vi "Job.BuildSpec_BuildSpecification.vi"(8 "error in (no error)":errorcluster, 11 "Job.BuildSpec in":refnum<class "Job.BuildSpec.lvclass">) -> (0 "error out":errorcluster, 3 "Job.BuildSpec out":refnum<class "Job.BuildSpec.lvclass">)   [LabVIEW 2013, in "Job.BuildSpec.lvclass"]
uses:
  Job.BuildSpec.lvclass
  Job.BuildSpec.lvclass/Job.BuildSpec.ctl
  <vilib>/AppBuilder/AB_API_Simple/Build (path).vi
  <vilib>/LabVIEW Open Source Project/Cron Scheduler/Job/Job.lvclass
  <vilib>/AppBuilder/AB_API_Simple/NI_App_Builder_API.lvlib
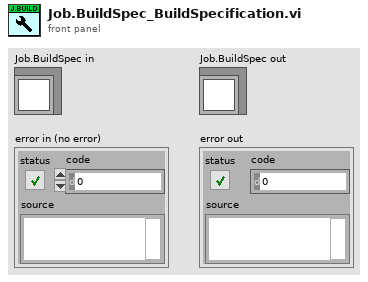
[diagram p1: front panel]
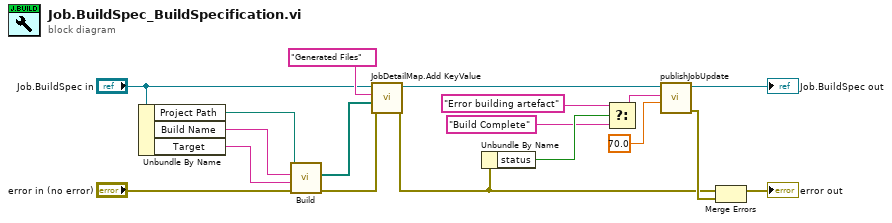
[diagram p0: block diagram]
diagram:
  n1 = Unbundle By Name("Job.BuildSpec in") -> ("Project Path"=w1:path, "Build Name"=w7:string, "Target"=w8:string)
  n2 = call-poly <vilib>:"Build.vi"("error in (no error)"="error in (no error)", "Name of target (My Computer)"=w8, "Name of build specification (if empty: build all)"=w7, "Path to project"=w1) -> ("error out"=w4:errorcluster, "Generated files"=w2:path[])  [unwired: 6 in]
  n3 = call <vilib>:"JobDetailMap.Add KeyValue.vi"("error in (no error)"=w4, "Value"=w2, "Key"="Generated Files", "Job in"="Job.BuildSpec in") -> ("error out"=w3:errorcluster, "Job out"=w5:refnum<class "Job.BuildSpec.lvclass">)  [unwired: 6 in]
  n4 = Unbundle By Name(w3) -> ("status"=w14:bool)
  n5 = Select(t="Error building artefact" ("Status Message"), s=w14, f="Build Complete" ("Status Message")) -> (s? t:f=w11:string)
  n6 = call <vilib>:"publishJobUpdate.vi"("% Complete (NaN if unknown)"=70.0, "Status Message"=w11, "Job in"=w5) -> ("error out"=w17:errorcluster, "Job out"=→"Job.BuildSpec out":refnum<class "Job.BuildSpec.lvclass">)  [unwired: 7 in]
  n7 = Merge Errors(w3, w17) -> (→"error out":errorcluster)
